vi "Umgebung.GetRef.vi"(8 "Error in":errorcluster) -> (0 "Error out":errorcluster, 3 "Umgebung":refnum<data-value>)   [LabVIEW 2016, in "Umgebung.lvclass"]
uses:
  Umgebung.lvclass
  Package ResourceControl/ObjectHandler/ObjectHandler.GetObjectWType.ctl
  Package ResourceControl/ObjectHandler/ObjectHandler.ObjectWType.ctl
  Package ResourceControl/ObjectHandler/ObjectHandler.ObjectType.ctl
  Package ResourceControl/ObjectHandler/ObjectHandler.lvclass
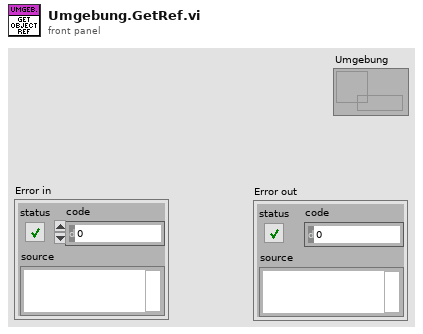
[diagram p1: front panel]
types:
  T1 = typedef "ObjectHandler.lvclass/ObjectHandler.GetObjectWType.ctl" = cluster{"Name":string, "Caller":string}
  T2 = typedef "ObjectHandler.lvclass/ObjectHandler.ObjectWType.ctl" = cluster{"ObjectType":T3, "Object":variant}
  T3 = typedef "ObjectHandler.lvclass/ObjectHandler.ObjectType.ctl" = enum16{"undefined", "ObjectHandler", "ViHandler", "ErrorHandler", "CentralStorage", "Hausmodell", "Sondenmodell", "Wärmepumpe", "Umgebung"}
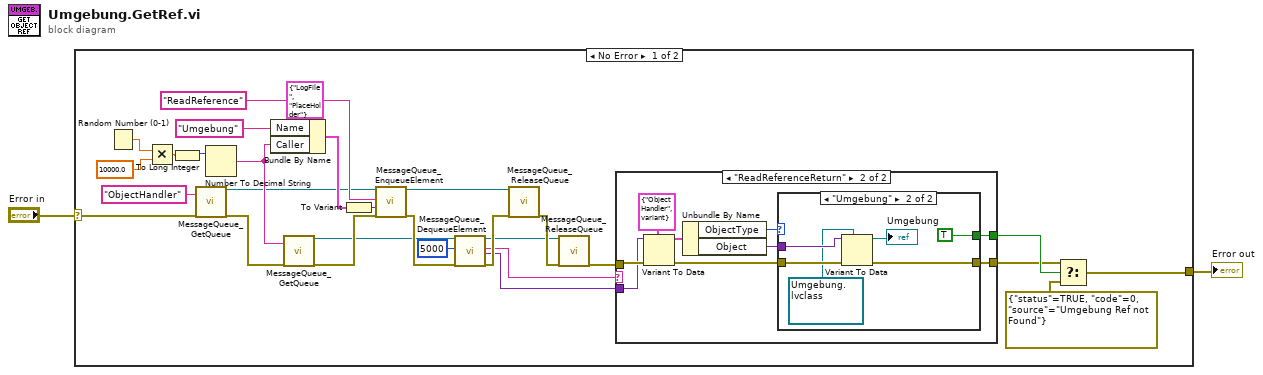
[diagram p0: block diagram]
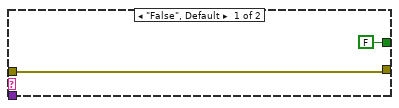
[diagram p2: hidden frame]
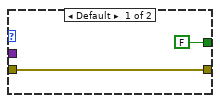
[diagram p3: hidden frame]
diagram:
  n1 = case shown="No Error" "Error in" {
    selector: "Error in" -> [w6 w51]
    tunnel: [w31 w51] -> w2
    frame No Error {
      n2 = Random Number (0-1)() -> (number: 0 to 1=w30:dbl)
      n3 = Multiply(x=w30, y=10000.0) -> (x*y=w28:dbl)
      n4 = To Long Integer(number=w28) -> (32bit integer=w27:i32)
      n5 = call "MessageQueue_GetQueue.vi"("Name"="ObjectHandler", "ErrorIn"=w6) -> ("QueueOut"=w4:refnum<queue>, "ErrorOut"=w3:errorcluster)  [unwired: 15 in, 1 out]
      n6 = Number To Decimal String(number=w27) -> (decimal integer string=w12:string)  [unwired: 1 in]
      n7 = Bundle By Name(cluster=T1 {"Name"="LogFile", "Caller"="PlaceHolder"} ("GetRefInput"), "Name"="Umgebung", "Caller"=w12) -> (w11:T1)
      n8 = call "MessageQueue_GetQueue.vi"("Name"=w12, "ErrorIn"=w3) -> ("QueueOut"=w21:refnum<queue>, "ErrorOut"=w26:errorcluster)  [unwired: 15 in, 1 out]
      n9 = To Variant(anything=w11) -> (Variant=w16:variant)
      n10 = call "MessageQueue_EnqueueElement.vi"("QueueIn"=w4, "Message"="ReadReference", "Data"=w16, "ErrorIn"=w26) -> ("QueueOut"=w22:refnum<queue>, "ErrorOut"=w25:errorcluster)  [unwired: 14 in]
      n11 = call "MessageQueue_DequeueElement.vi"("QueueIn"=w21, "Timeout"=5000, "ErrorIn"=w25) -> ("QueueOut"=w20:refnum<queue>, "Message"=w18:string, "Data"=w14:variant, "ErrorOut"=w24:errorcluster)  [unwired: 12 in, 1 out]
      n12 = call "MessageQueue_ReleaseQueue.vi"("QueueIn"=w22, "ErrorIn"=w24) -> ("ErrorOut"=w23:errorcluster)  [unwired: 15 in, 2 out]
      n13 = call "MessageQueue_ReleaseQueue.vi"("QueueIn"=w20, "ErrorIn"=w23) -> ("ErrorOut"=w15:errorcluster)  [unwired: 15 in, 2 out]
      n14 = case shown="\"ReadReferenceReturn\"" w18 {
        tunnel: w15 -> [w32 w42]
        tunnel: w14 -> [_ w41]
        tunnel: [w32 w35] -> w9
        tunnel: [FALSE w34] -> w10
        frame "False", Default {
        }
        frame "ReadReferenceReturn" {
          n15 = Variant To Data(error in=w42, type=T2 {"ObjectType"=enum."ObjectHandler", "Object"=variant} ("ObjectWType"), Variant=w41) -> (data=w39:T2, error out=w36:errorcluster)
          n16 = Unbundle By Name(w39) -> ("ObjectType"=w38:T3, "Object"=w37:variant)
          n17 = case shown="\"Umgebung\"" w38 {
            tunnel: w37 -> [_ w50]
            tunnel: w36 -> [w44 w49]
            tunnel: [w44 w48] -> w35
            tunnel: [FALSE TRUE] -> w34
            frame Default {
            }
            frame "Umgebung" {
              n18 = Variant To Data(error in=w49, type=refnum<data-value> refnum ("data value reference"), Variant=w50) -> (data=→"Umgebung":refnum<data-value>, error out=w48:errorcluster)
            }
          }
        }
      }
      n19 = Select(t=w9, s=w10, f=errorcluster {"status"=TRUE, "code"=0, "source"="Umgebung Ref not Found"}) -> (s? t:f=w31:errorcluster)
    }
    frame Error {
    }
  }
  "Error out" <- w2
